vi "Convert_Version_Info.vi"(8 "error in (no error)":errorcluster, 11 "AB_Build in":refnum<class "AB_Build.lvclass">) -> (0 "error out":errorcluster, 2 "input version info":T1={"PrivateBuild"="", "SpecialBuild"="", "LegalCopyright"="", "LegalTrademarks"="", "Comments"="", "FileDescription"="", "InternalName"="", "file version"={"major"=1, "minor"=0, "patch"=0, "build"=0}, "ProductName"="", "FileType"=0, "CompanyName"="", "OriginalFilename"=""} {"FileType" items=["VFT_UNKNOWN", "VFT_APP", "VFT_DLL", "VFT_DRV", "VFT_FONT", "VFT_VXD", "-", "VFT_STATIC_LIB"]}, 3 "AB_Build out":refnum<class "AB_Build.lvclass">)   [LabVIEW 2020, in "AB_Build.lvclass"]
uses:
  <vilib>/AppBuilder/AB_Classes/Build/AB_Build.lvclass
  <vilib>/AppBuilder/AB_Version_Info.ctl
  <vilib>/AppBuilder/AB_Classes/Build/AB_Build.lvclass/AB_Build.ctl
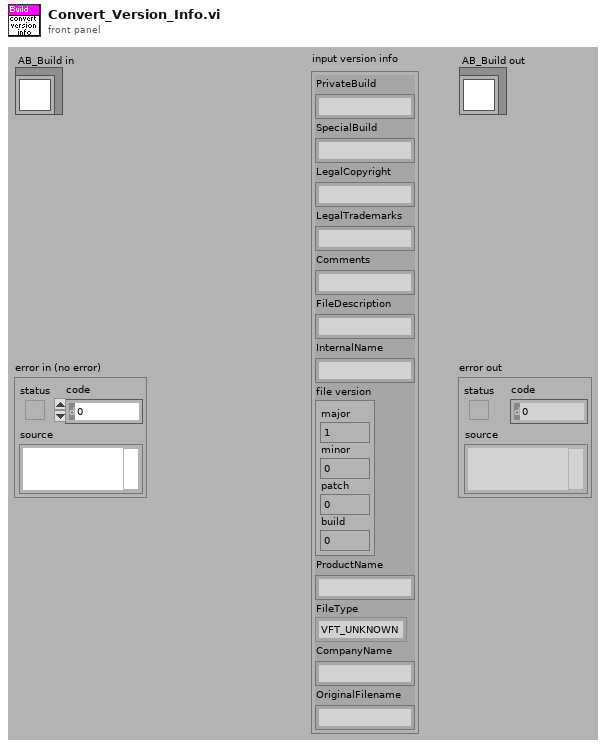
[diagram p1: front panel]
types:
  T1 = typedef "AB_Version_Info.ctl" = cluster{"PrivateBuild":string, "SpecialBuild":string, "LegalCopyright":string, "LegalTrademarks":string, "Comments":string, "FileDescription":string, "InternalName":string, "file version":cluster{"major":u16, "minor":u16, "patch":u16, "build":u16}, "ProductName":string, "FileType":u16, "CompanyName":string, "OriginalFilename":string}
  T2 = cluster{"major":u16, "minor":u16, "patch":u16, "build":u16}
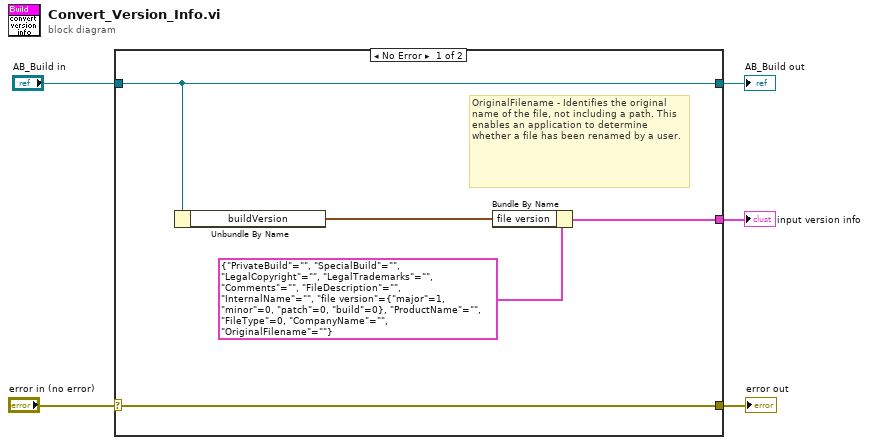
[diagram p0: block diagram]
diagram:
  n1 = case shown="No Error" "error in (no error)" {
    selector: "error in (no error)" -> [w10 w12]
    tunnel: [w10 w12] -> w4
    tunnel: [w9 w11] -> w2
    tunnel: "AB_Build in" -> [w9 w11]
    tunnel: [w6 _] -> w1
    frame No Error {
      # "OriginalFilename - Identifies the original name of the file, not including a path. This enables an application to determine whether a file has been renamed by a user."
      n2 = Unbundle By Name(w9) -> ("buildVersion"=w7:T2)
      n3 = Bundle By Name(cluster=T1 {"PrivateBuild"="", "SpecialBuild"="", "LegalCopyright"="", "LegalTrademarks"="", "Comments"="", "FileDescription"="", "InternalName"="", "file version"={"major"=1, "minor"=0, "patch"=0, "build"=0}, "ProductName"="", "FileType"=0, "CompanyName"="", "OriginalFilename"=""} ("input version info"), "file version"=w7) -> (w6:T1)
    }
    frame Error {
    }
  }
  "error out" <- w4
  "AB_Build out" <- w2
  "input version info" <- w1
